vi "Remove Line.vi"(8 "error in":errorcluster, 10 "Active Line Name":string, 11 "Objects":T1) -> (0 "error out":errorcluster)   [LabVIEW 2017, in "JSON_RPC_Interface editor node.lvclass"]
doc: "This VI will remove a line from the configuration and disconect any tag connected to the channels in the line"
uses:
  JSON_RPC_Interface editor node.lvclass
  <vilib>/NI/DCAF/Tag Editor Core/Table API/Table Manager/object ref.ctl
  <vilib>/NI/DCAF/Tag Editor Core/Configuration Editor/Classes/Engine Parent/Engine Parent Editor Node.lvclass
  <vilib>/NI/DCAF/Tag Editor Core/Configuration Editor/Classes/Module editor node/module editor node.lvclass
  module/configuration/JSON_RPC_Interface configuration.lvclass
  C:/Program Files (x86)/National Instruments/LabVIEW 2017/vi.lib/NI/Configuration Framework/serializable configuration/NISE_CEF_serializable configuration.lvclass
  <vilib>/NI/Configuration Framework/serializable configuration/NISE_CEF_serializable configuration.lvclass/NISE_CEF_serializable configuration.ctl
  <vilib>/Utility/LVClass/Get LV Class Name.vi
  <vilib>/NI/Configuration Framework/error generator/NISE_error generator.vi
  <vilib>/NI/Configuration Framework/serializable configuration/NISE_CEF_serializable configuration.lvclass
  <vilib>/NI/DCAF/Tag Editor Core/Table API/Table Manager/Table Manager.lvclass
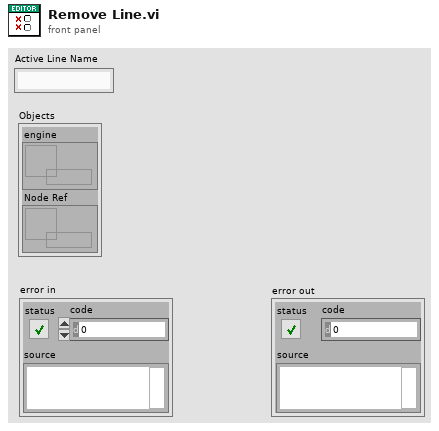
[diagram p1: front panel]
types:
  T1 = typedef "Table Manager.lvlib/Table Manager.lvclass/object ref.ctl" = cluster{"engine":refnum<data-value>, "Node Ref":refnum<data-value>}
  T2 = typedef "JSON_RPC_Interface configuration.lvclass/Line.ctl" = cluster{"channel":refnum<class "TBM channel.lvclass">}
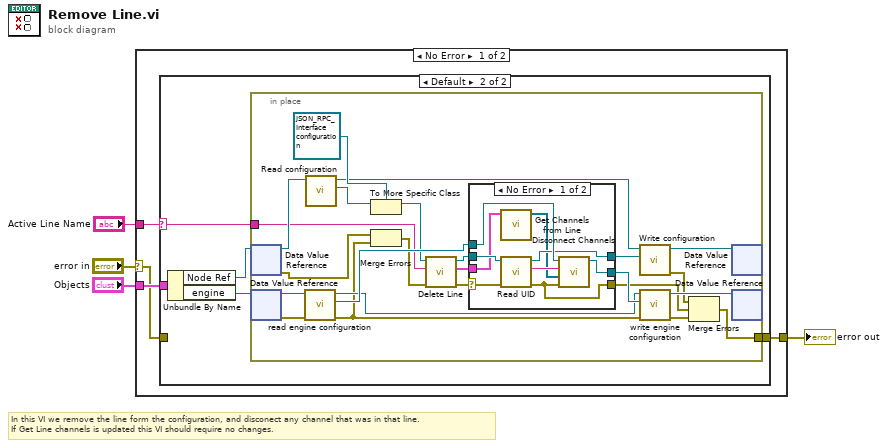
[diagram p0: block diagram]
diagram:
  # "In this VI we remove the line form the configuration, and disconect any channel that was in that line.\nIf Get Line channels is updated this VI should require no changes."
  n1 = case shown="No Error" "error in" {
    selector: "error in" -> [w5 w51]
    tunnel: "Objects" -> [w7 _]
    tunnel: [w8 w51] -> w3
    tunnel: "Active Line Name" -> [w6 _]
    frame No Error {
      n2 = case shown="Default" w6 {
        selector: w6 -> [_ w10]
        tunnel: [w9 w14] -> w8
        tunnel: w7 -> [_ w13]
        tunnel: w5 -> [w9 _]
        frame " " {
        }
        frame Default {
          n3 = Unbundle By Name(w13) -> ("Node Ref"=w11:refnum<data-value>, "engine"=w12:refnum<data-value>)
          n4 = in-place {
            in-place-border: [w17] -> w14
            in-place-border: w10 -> [w24]
            n5 = in-place-dvr #1(w11) -> (w30:refnum<class "module editor node.lvclass">, w31:errorcluster)
            n6 = in-place-dvr #2(w12) -> (w36:refnum<class "Engine Parent Editor Node.lvclass">, w35:errorcluster)
            n7 = call <vilib>:"read engine configuration.vi"("error in"=w35, "Engine Parent Editor Node in"=w36) -> ("error out"=w32:errorcluster, "engine configuration"=w34:refnum<class "engine configuration.lvclass">, "Engine Parent Editor Node out"=w33:refnum<class "Engine Parent Editor Node.lvclass">)  [unwired: 7 in]
            n8 = call-dynamic "Read configuration.vi"("NISE_CEF_serializable node in"=w30) -> ("configuration"=w28:refnum<class "NISE_CEF_serializable configuration.lvclass">, "NISE_CEF_serializable node out"=w26:refnum<class "module editor node.lvclass">)  [unwired: 8 in, 1 out]
            n9 = To More Specific Class(target class=refnum<class "JSON_RPC_Interface configuration.lvclass"> refnum ("tag bus configurable plugin module configuration out"), reference=w28) -> (specific class reference=w23:refnum<class "JSON_RPC_Interface configuration.lvclass">)  [unwired: 1 in, 1 out]
            n10 = Merge Errors(w31, w32) -> (w21:errorcluster)
            n11 = call "Delete Line.vi"("error in"=w21, "Line Name"=w24, "JSON_RPC_Interface configuration in"=w23) -> ("error out"=w20:errorcluster, "Deleted Line"=w15:T2, "JSON_RPC_Interface configuration out"=w22:refnum<class "JSON_RPC_Interface configuration.lvclass">)  [unwired: 6 in]
            n12 = case shown="No Error" w20 {
              selector: w20 -> [w42 w48]
              tunnel: w22 -> [w45 w49]
              tunnel: w34 -> [w47 w50]
              tunnel: [w46 w50] -> w37
              tunnel: [w43 w49] -> w25
              tunnel: [w39 w48] -> w16
              tunnel: w15 -> [w41 _]
              frame No Error {
                n13 = call "Get Channels from Line.vi"("Line"=w41) -> ("Channels"=w40:refnum<class "TBM channel.lvclass">[])  [unwired: 10 in]
                n14 = call <vilib>:"Read UID.vi"("error in"=w42, "configuration in"=w45) -> ("error out"=w39:errorcluster, "instance id"=w44:string, "configuration out"=w43:refnum<class "JSON_RPC_Interface configuration.lvclass">)  [unwired: 7 in]
                n15 = call "Disconnect Channels.vi"("error in (no error)"=w39, "Deleted Channels"=w40, "instance id"=w44, "Engine Configuration in"=w47) -> ("Engine Configuration out"=w46:refnum<class "engine configuration.lvclass">)  [unwired: 6 in, 1 out]
              }
              frame Error {
              }
            }
            n16 = call-dynamic "Write configuration.vi"("configuration"=w25, "NISE_CEF_serializable node in"=w26) -> ("error out"=w19:errorcluster, "NISE_CEF_serializable node out"=w27:refnum<class "module editor node.lvclass">)  [unwired: 8 in]
            n17 = call <vilib>:"write engine configuration.vi"("error in"=w32, "engine configuration"=w37, "Engine Parent Editor Node in"=w33) -> ("error out"=w18:errorcluster, "Engine Parent Editor Node out"=w38:refnum<class "Engine Parent Editor Node.lvclass">)  [unwired: 7 in]
            n18 = Merge Errors(w19, w16, w18) -> (w17:errorcluster)
            n19 = in-place-dvr #1(w27) -> ()  [unwired: 2 out]
            n20 = in-place-dvr #2(w38) -> ()  [unwired: 2 out]
          }
        }
      }
    }
    frame Error {
    }
  }
  "error out" <- w3
